vi "BackEvent_ZA.vi"(8 "error in (no error)":errorcluster, 10 "Back":bool, 11 "Zen Analytics in":refnum<class "Zen Analytics.lvclass">) -> (0 "error out":errorcluster, 3 "Zen Analytics out":refnum<class "Zen Analytics.lvclass">)   [LabVIEW 2015, in "Zen Analytics.lvclass"]
uses:
  Zen Analytics.lvclass
  Zen Analytics.lvclass/Zen Analytics.ctl
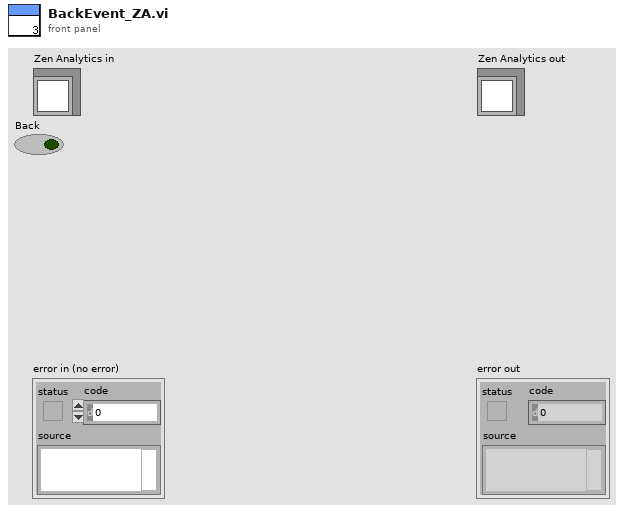
[diagram p1: front panel]
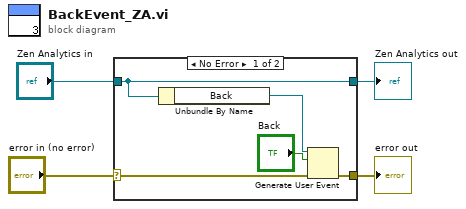
[diagram p0: block diagram]
diagram:
  n1 = case shown="No Error" "error in (no error)" {
    selector: "error in (no error)" -> [w6 w11]
    tunnel: [w5 w11] -> w3
    tunnel: [w9 w10] -> w1
    tunnel: "Zen Analytics in" -> [w9 w10]
    frame No Error {
      n2 = Unbundle By Name(w9) -> ("Back"=w8:refnum<user-event>)
      n3 = Generate User Event(user event=w8, event data cluster="Back", error in=w6) -> (error out=w5:errorcluster)  [unwired: 1 in, 1 out]
    }
    frame Error {
    }
  }
  "error out" <- w3
  "Zen Analytics out" <- w1
